vi "Stop Core.vi"(10 "final error code":i32, 11 "FirstAF in":refnum<class "FirstAF.lvclass">) -> (3 "FirstAF out":refnum<class "FirstAF.lvclass">)   [LabVIEW 2019, in "FirstAF.lvlib" / "FirstAF.lvclass"]
doc: "(<B>Filename</B>: Actor Framework.lvlib:Actor.lvclass:Stop Core.vi)\n\nDefines what the actor does before it stops. Use the <B>final error code</B> input to determine whether the actor shut down in response to an error.\n\nBy default, this method passes the Stop message along to all auto-stop nested actors. A descendant class may override this method to define additional behavior, such as shutting down any processes the actor initiated in its override of the Actor Core method."
uses:
  FirstAF.lvclass
  FirstAF.lvclass/FirstAF.ctl
  <vilib>/ActorFramework/Actor/Actor.lvclass
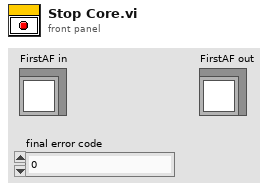
[diagram p1: front panel]
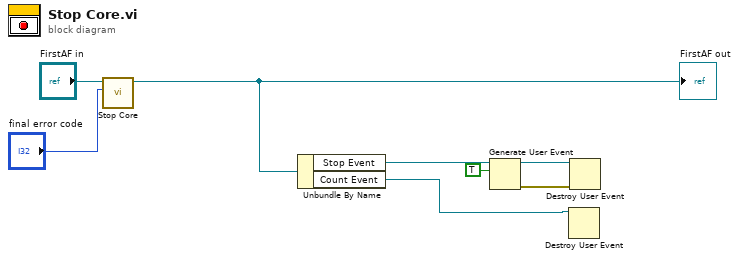
[diagram p0: block diagram]
diagram:
  n1 = call-parent "Stop Core.vi"("final error code"="final error code", "Actor in"="FirstAF in") -> ("Actor out"=w6:refnum<class "FirstAF.lvclass">)  [unwired: 9 in]
  "FirstAF out" <- w6
  n2 = Unbundle By Name(w6) -> ("Stop Event"=w5:refnum<user-event>, "Count Event"=w2:refnum<user-event>)
  n3 = Generate User Event(user event=w5, event data cluster=TRUE ("event data")) -> (user event out=w4:refnum<user-event>, error out=w3:errorcluster)  [unwired: 2 in]
  n4 = Destroy User Event(user event=w2) -> ()  [unwired: 1 in, 1 out]
  n5 = Destroy User Event(user event=w4, error in=w3) -> ()  [unwired: 1 out]
